vi "Fixed Frequency Player.vi"() -> ()   [LabVIEW 2016]
uses:
  <vilib>/sound2/lvsound2.llb/Sound Data Format.ctl
  <vilib>/Platform/TimedLoop/XDataNode/timing_clust.ctl
  <vilib>/Platform/TimedLoop/XDataNode/nitl_modes.ctl
  <vilib>/Platform/TimedLoop/XDataNode/wakeup.ctl
  <vilib>/express/express analysis/Spectral/Block/exnSpectralBlock spectral measurements RMS poly.vi
  <vilib>/express/express analysis/Spectral/Block/exnSpectralBlock spectral measurements RMS WFM.vi
  <vilib>/sound2/lvsound2.llb/Sound Output Write (DBL Single).vi
  <vilib>/Platform/TimedLoop/XDataNode/XDataNode.xnode
  <vilib>/express/express analysis/Spectral/XNode/ExpressSpectralMeasurementsBlockNode.xnode
  <vilib>/measure/NI_MABase.lvlib
  <vilib>/Platform/TimedLoop/XDataNode/XDNodeRunTimeDep.lvlib
panel:
  in  "Noise Amplitude":dbl(slide)=0.5 caption="Amplitude" min=0.0 max=1.0 scale=0.0..1.0
  in  "Signal Amplitude":dbl(slide)=0.5 caption="Amplitude" min=0.0 max=1.0 scale=0.0..1.0
  in  "device ID":u32
  out "Frequency Domain Signal":cluster{"f0":dbl, "df":dbl, "magnitude":dbl[]}(graph)
  out "Time Domain Signal":waveform(dbl)(graph) caption="Sine"
  in  "Signal Frequency":dbl(slide)=400.0 caption="Frequency" min=1.0 max=20000.0 scale=1.0..20000.0
  in  "Signal Offset":dbl caption="Offset"
  in  "Signal Phase":dbl caption="Phase"
  in  "Select Noise":u16(ring) items=["No Noise", "White Noise (uniform)", "Pink Noise (1/f)"]
  in  "Select Filter":u16(ring) items=["No Filter", "Smoothing", "Highpass", "Lowpass", "Bandpass"]
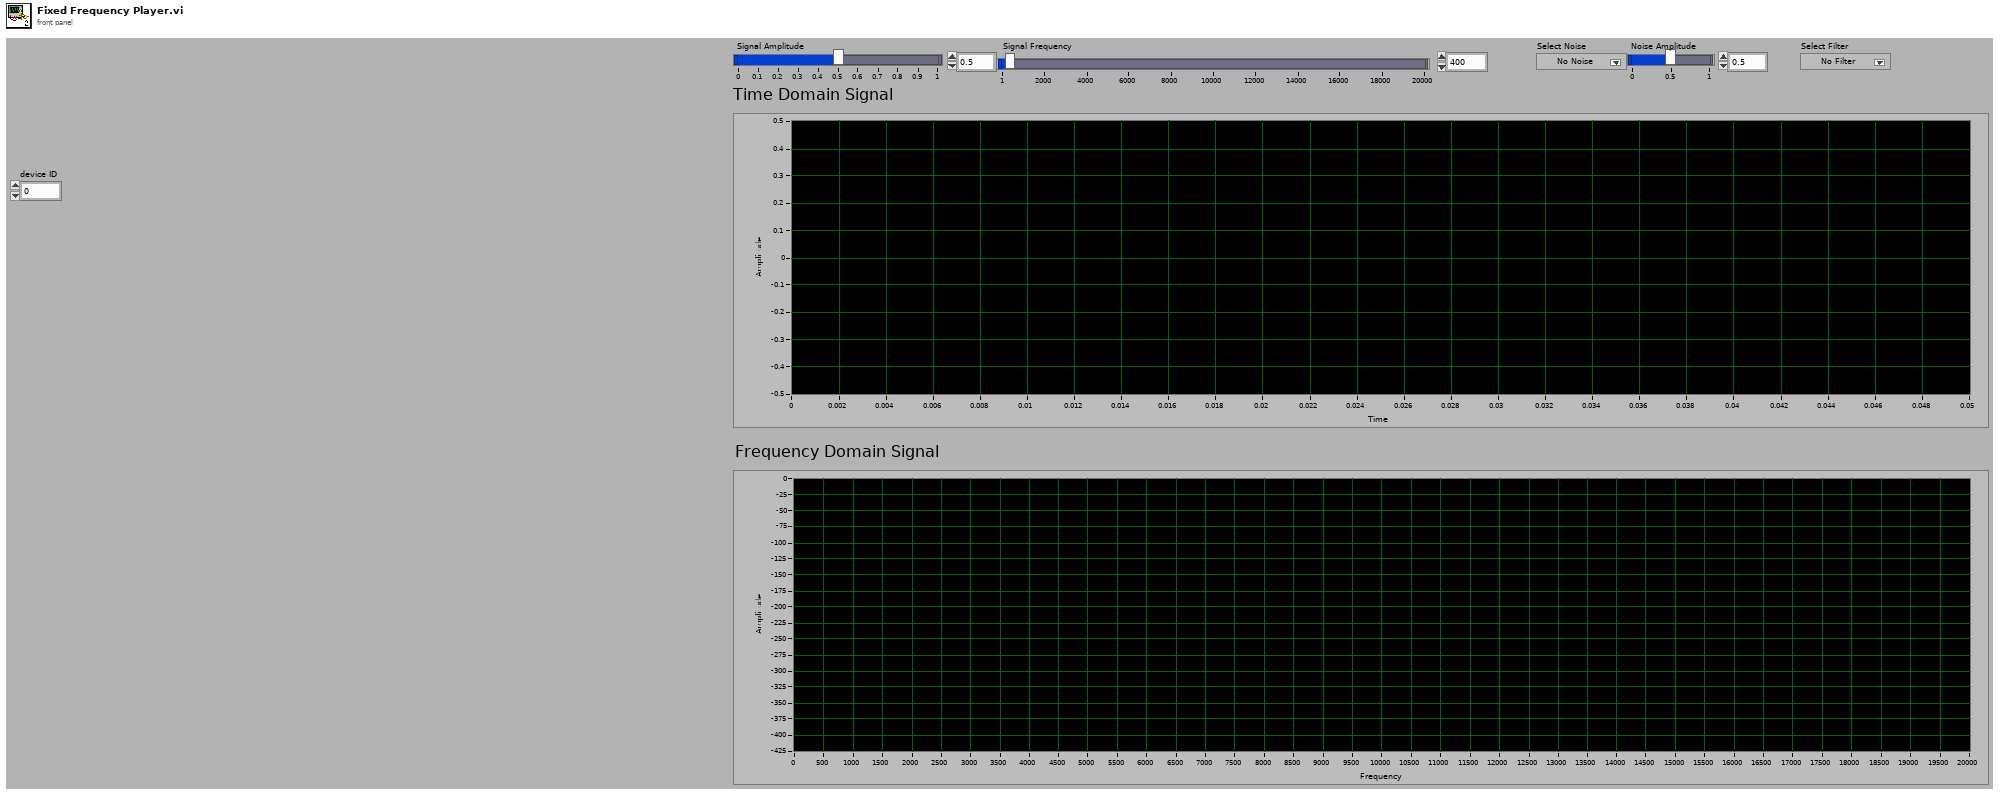
[diagram p1: front panel]
types:
  T1 = typedef "Sound Data Format.ctl" = cluster{"sample rate (S/s)":dbl, "number of channels":i32, "bits per sample":i32}
  T2 = typedef "Sound Output Task ID.ctl" = u32
  T3 = cluster{"sample rate (S/s)":dbl, "sample rate (S/s)":dbl}
  T4 = typedef "XDNodeRunTimeDep.lvlib/timing_clust.ctl" = cluster{"Expected End [f-1]":u64, "Actual End [f-1]":u64, "Finished Late? [f-1]":bool, "Expected End [i-1]":u64, "Actual End [i-1]":u64, "Finished Late? [i-1]":bool, "Expected Start [i]":u64, "Actual Start [i]":u64, "Expected Start [f]":u64, "Actual Start [f]":u64, "Source Name":string, "Structure Name":string, "Period":i64, "Deadline":i64, "Offset":i64, "Start":i64, "Priority":i32, "Timeout":i32, "Mode":T5, "Wakeup Reason":T6, "Error":errorcluster, "Source Type":string, "Secondary Source Type":string, "Global End Time":u64, "Global Start Time":u64, "Frame Duration":u64, "Iteration Duration":u64, "Assigned CPU":i32, "I/O Scan Engine Mode":u32}
  T5 = typedef "XDNodeRunTimeDep.lvlib/nitl_modes.ctl" = enum32{"No Change", "Process missed periods, maintain original phase", "Discard missed periods, maintain original phase", "Process missed periods, ignore original phase", "Discard missed periods, ignore original phase"}
  T6 = typedef "XDNodeRunTimeDep.lvlib/wakeup.ctl" = enum32{"Normal", "Aborted", "Asynchronous wakeup", "Timing source error", "Timed loop error", "Timeout"}
  T7 = cluster{"lower cutoff freq":dbl, "higher cutoff freq":dbl, "order":i32}
  T8 = cluster{"averaging mode":u16, "weighting mode":u16, "number of averages":u32}
  T9 = cluster{"dB On (F)":bool, "unwrap phase (F)":bool, "convert to degree (F)":bool}
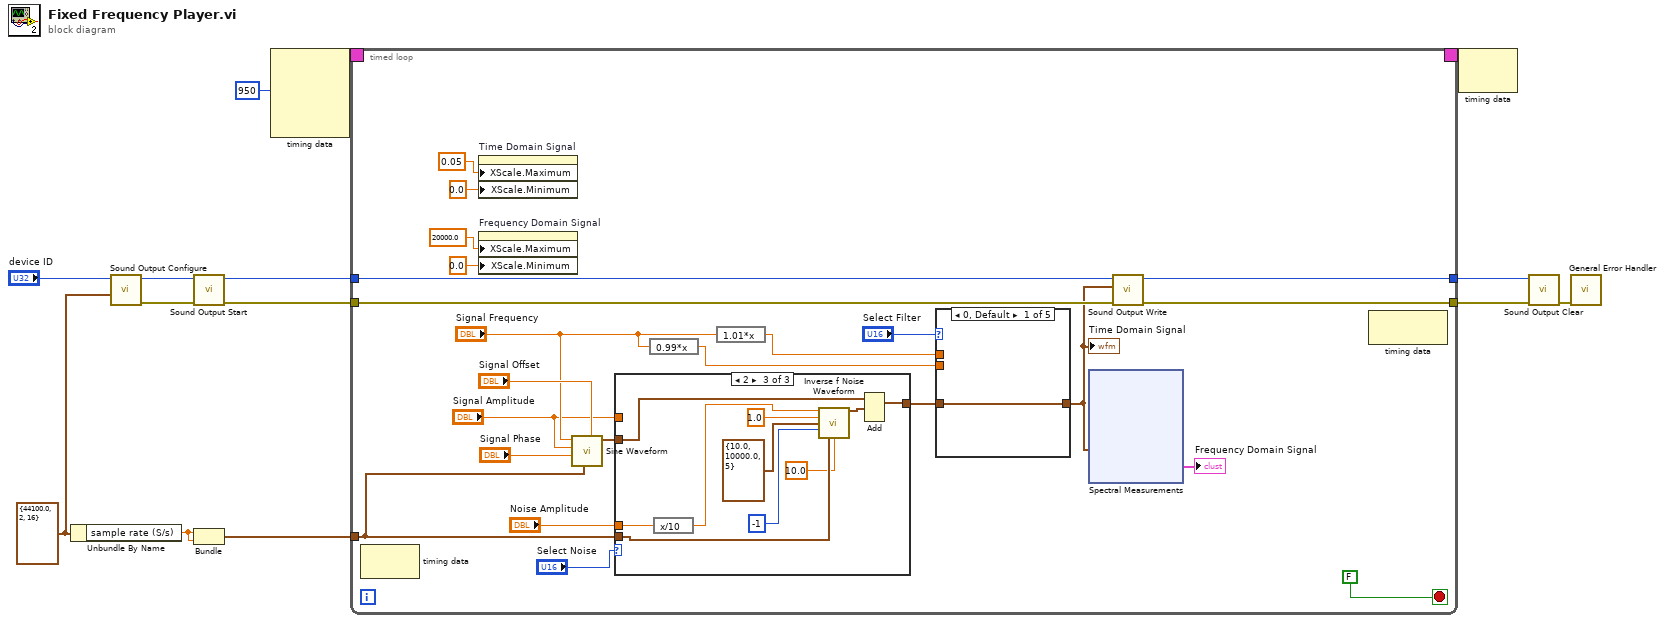
[diagram p0: block diagram]
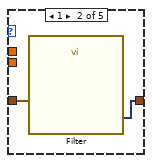
[diagram p2: hidden frame]
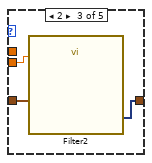
[diagram p3: hidden frame]
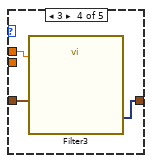
[diagram p4: hidden frame]
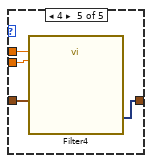
[diagram p5: hidden frame]
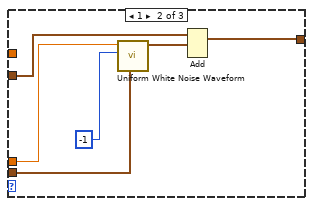
[diagram p7: hidden frame]
diagram:
  w11 = T1 {"sample rate (S/s)"=44100.0, "number of channels"=2, "bits per sample"=16} ("sound format")
  n1 = Unbundle By Name(w11) -> ("sample rate (S/s)"=w2:dbl)
  n2 = call <vilib>:"Sound Output Configure.vi"("sound format"=w11, "device ID"="device ID") -> ("error out"=w12:errorcluster, "task ID"=w13:T2)  [unwired: 8 in]
  n3 = call <vilib>:"Sound Output Start.vi"("error in (no error)"=w12, "task ID"=w13) -> ("error out"=w8:errorcluster, "task ID out"=w9:T2)  [unwired: 8 in]
  n4 = Bundle("sample rate (S/s)"=w2, "sample rate (S/s)"=w2) -> (w1:T3)  [unwired: 1 in]
  n5 = node-c288(i64 950 ("Period")) -> (w5:T4)  [unwired: 3 in]
  n6 = timed-loop {
    tunnel: w9 -> [w22]
    tunnel: w8 -> [w21]
    tunnel: [w20] -> w7
    tunnel: [w19] -> w6
    timing: w5 -> [_]
    timing-out: [_] -> w4
    tunnel: w1 -> [w15]
    stop <- FALSE stop-if-true
    n7 = node-c288() -> ()  [unwired: 1 in, 1 out]
    n8 = property on="Time Domain Signal" class="WFGraph (strict)"("XScale.Maximum"=0.05 ("X Scale.Range:Maximum"), "XScale.Minimum"=0.0 ("X Scale.Range:Minimum")) -> ()  [unwired: 2 in, 2 out]
    n9 = property on="Frequency Domain Signal" class="WFGraph (strict)"("XScale.Maximum"=20000.0 ("X Scale.Range:Maximum"), "XScale.Minimum"=0.0 ("X Scale.Range:Minimum")) -> ()  [unwired: 2 in, 2 out]
    n10 = call <vilib>:"Sine Waveform.vi"("offset"="Signal Offset", "sampling info"=w15, "phase"="Signal Phase", "amplitude"="Signal Amplitude", "frequency"="Signal Frequency") -> ("signal out"=w31:waveform(dbl))  [unwired: 5 in, 1 out]
    n11 = case shown="2" "Select Noise" {
      tunnel: [w53 w58 w67] -> w26
      tunnel: w31 -> [w53 w59 w69]
      tunnel: "Signal Amplitude" -> [_ _ _]
      tunnel: w15 -> [_ w55 w64]
      tunnel: "Noise Amplitude" -> [_ w54 w61]
      frame 0, Default {
      }
      frame 1 {
        n12 = call <vilib>:"Uniform White Noise Waveform.vi"("sampling info"=w55, "seed"=-1, "amplitude"=w54) -> ("signal out"=w57:waveform(dbl))  [unwired: 7 in, 1 out]
        n13 = Add(1:w57, 2:w59) -> (0:w58:waveform(dbl))  [unwired: 1 in, 1 out]
      }
      frame 2 {
        n14 = expression code="x/10"(w61) -> (w60:dbl)
        n15 = call <vilib>:"Inverse f Noise Waveform.vi"("noise density"=w60, "exponent"=1.0, "filter specifications"=T7 {"lower cutoff freq"=10.0, "higher cutoff freq"=10000.0, "order"=5}, "seed"=-1, "sampling info"=w64, "reference freq (Hz)"=10.0) -> ("signal out"=w68:waveform(dbl))  [unwired: 5 in, 4 out]
        n16 = Add(1:w68, 2:w69) -> (0:w67:waveform(dbl))  [unwired: 1 in, 1 out]
      }
    }
    n17 = expression code="0.99*x"("Signal Frequency") -> (w29:dbl)
    n18 = expression code="1.01*x"("Signal Frequency") -> (w27:dbl)
    n19 = case shown="0, Default" "Select Filter" {
      tunnel: [w40 w41 w44 w47 w49] -> w18
      tunnel: w26 -> [w40 w42 w45 w48 w50]
      tunnel: w29 -> [_ _ w43 _ w51]
      tunnel: w27 -> [_ _ _ w46 w52]
      frame 0, Default {
      }
      frame 1 {
        n20 = call "Filter"("Signal"=w42) -> ("Filtered Signal"=w41:dynamicdata)  [unwired: 9 in, 1 out]
      }
      frame 2 {
        n21 = call "Filter2"("Lower Cut-Off"=w43, "Signal"=w45) -> ("Filtered Signal"=w44:dynamicdata)  [unwired: 8 in, 1 out]
      }
      frame 3 {
        n22 = call "Filter3"("Lower Cut-Off"=w46, "Signal"=w48) -> ("Filtered Signal"=w47:dynamicdata)  [unwired: 8 in, 1 out]
      }
      frame 4 {
        n23 = call "Filter4"("Lower Cut-Off"=w51, "Upper Cut-Off"=w52, "Signal"=w50) -> ("Filtered Signal"=w49:dynamicdata)  [unwired: 7 in, 1 out]
      }
    }
    "Time Domain Signal" <- w18
    n24 = xnode "Spectral Measurements"("Signals"=w18) -> ("FFT - (RMS)"=→"Frequency Domain Signal":cluster{"f0":dbl, "df":dbl, "magnitude":dbl[]})  [unwired: 1 in, 2 out]
    n25 = call-poly <vilib>:"Sound Output Write.vi"("error in (no error)"=w21, "data"=w18, "task ID"=w22) -> ("error out"=w19:errorcluster, "task ID out"=w20:T2)  [unwired: 7 in]
    n26 = node-c288() -> ()  [unwired: 1 in, 1 out]
  }
  n27 = node-c288(w4) -> ()  [unwired: 1 out]
  n28 = call <vilib>:"Sound Output Clear.vi"("error in (no error)"=w6, "task ID"=w7) -> ("error out"=w10:errorcluster)  [unwired: 9 in]
  n29 = call <vilib>:"General Error Handler.vi"("error in (no error)"=w10) -> ()  [unwired: 2 in, 13 out]
